vi "Init_GBL_Constant.vi"(8 "error in (no error)":errorcluster) -> (0 "error out":errorcluster)   [LabVIEW 2017]
doc: "Initialise Global variables and constants"
uses:
  <vilib>/Analysis/coordinate.llb/Wrap Angle (scalar).vi
  GBL/GBL_variables.vi
  <vilib>/Analysis/NI_AAL_Angle.lvlib
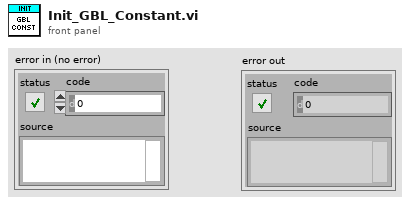
[diagram p1: front panel]
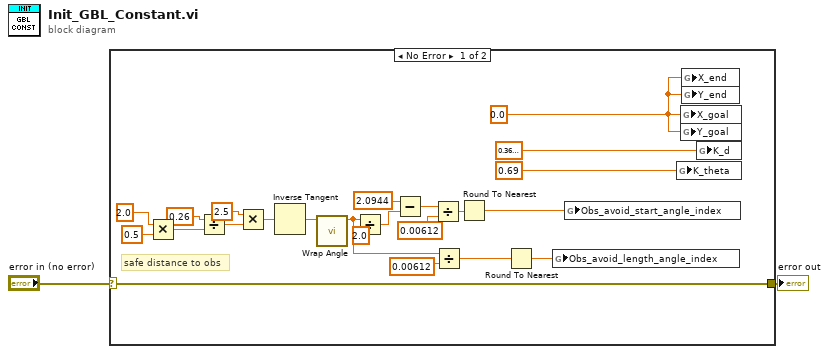
[diagram p0: block diagram]
diagram:
  n1 = case shown="No Error" "error in (no error)" {
    selector: "error in (no error)" -> [w24 w26]
    tunnel: [w24 w26] -> w1
    frame No Error {
      w4 = 0.0 ("X_goal")
      # "safe distance to obs"
      n2 = Multiply(x=2.0, y=0.5) -> (x*y=w8:dbl)
      n3 = Divide(x=0.26, y=w8) -> (x/y=w9:dbl)
      n4 = Multiply(x=2.5, y=w9) -> (x*y=w11:dbl)
      n5 = Inverse Tangent(1:w11) -> (0:w12:dbl)
      n6 = call-poly <vilib>:"Wrap Angle.vi"("angle in"=w12) -> ("angle out"=w16:dbl)  [unwired: 9 in, 1 out]
      n7 = Divide(x=w16, y=2.0) -> (x/y=w18:dbl)
      n8 = Subtract(x=2.0944, y=w18) -> (x-y=w22:dbl)
      n9 = Divide(x=w22, y=0.00612) -> (x/y=w20:dbl)
      n10 = Divide(x=w16, y=0.00612) -> (x/y=w15:dbl)
      n11 = Round To Nearest(number=w20) -> (nearest integer value=w14:dbl)
      n12 = Round To Nearest(number=w15) -> (nearest integer value=w13:dbl)
      n13 = global write "GBL_variables.vi" "Obs_avoid_length_angle_index"(w13) -> ()
      n14 = global write "GBL_variables.vi" "Obs_avoid_start_angle_index"(w14) -> ()
      n15 = global write "GBL_variables.vi" "K_theta"(0.69 ("K_theta")) -> ()
      n16 = global write "GBL_variables.vi" "X_goal"(w4) -> ()
      n17 = global write "GBL_variables.vi" "Y_goal"(w4) -> ()
      n18 = global write "GBL_variables.vi" "X_end"(w4) -> ()
      n19 = global write "GBL_variables.vi" "Y_end"(w4) -> ()
      n20 = global write "GBL_variables.vi" "K_d"(0.36000000000000004 ("K_d")) -> ()
    }
    frame Error {
    }
  }
  "error out" <- w1
